vi "Read Tag Data.vi"(8 "error in (no error)":errorcluster, 11 "Task D-O Channels":string[][](array[string])) -> (0 "error out":errorcluster, 3 "Array":bool[][](array[boolean]))   [LabVIEW 2018, in "DAQ.lvlib"]
uses:
  DAQ.lvlib
  Tag VIs/Tag FGV Operation Enum.ctl
  Shared Variables/Dynamic Shared Variables.lvlib
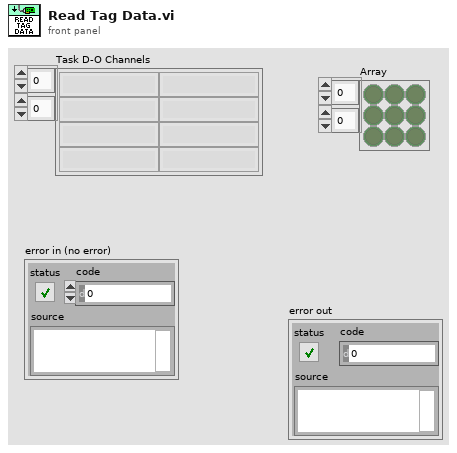
[diagram p1: front panel]
types:
  T1 = typedef "Tag FGV Operation Enum.ctl" = enum16{"Init", "Set Notification Queue", "Create Tag", "Commit", "Write Tag (Numeric)", "Write Tag (Boolean)", "Read All Tags", "Read One Tag", "Delete Tag Category", "Set Alarm Parameters (Numeric)", "Set Alarm Parameters (Boolean)", "Enable All Alarms", "Disable All Alarms", "Delete All Tags", "Read Alarms", "Ack Alarm"}
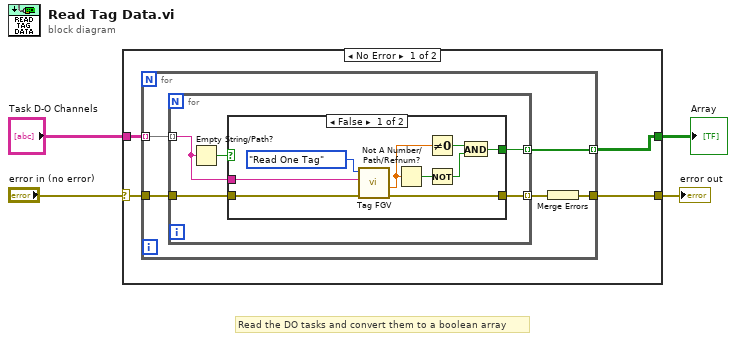
[diagram p0: block diagram]
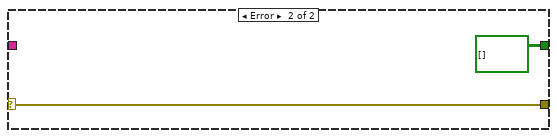
[diagram p3: hidden frame]
diagram:
  # "Read the DO tasks and convert them to a boolean array"
  n1 = case shown="No Error" "error in (no error)" {
    selector: "error in (no error)" -> [w6 w30]
    tunnel: [w8 w30] -> w4
    tunnel: "Task D-O Channels" -> [w7 _]
    tunnel: [w5 bool[][] []] -> w2
    frame No Error {
      n2 = for {
        tunnel: [w13] -> w8
        tunnel: w7 -> [w9] mode=indexing
        tunnel: w6 -> [w11]
        tunnel: [w10] -> w5 mode=indexing
        n3 = for {
          tunnel: [w16] -> w10 mode=indexing
          tunnel: w9 -> [w14] mode=indexing
          tunnel: w11 -> [w18]
          tunnel: [w17] -> w12 mode=indexing
          n4 = Empty String/Path?(string/path=w14) -> (empty?=w15:bool)
          n5 = case shown="False" w15 {
            tunnel: w14 -> [w26 _]
            tunnel: w18 -> [w25 w28]
            tunnel: [w24 w28] -> w17
            tunnel: [w22 _] -> w16
            frame False {
              n6 = call "Tag FGV.vi"("error in (no error)"=w25, "Tag Name"=w26, "Operation"=Tag_FGV_Operation_Enum."Read One Tag") -> ("error out"=w24:errorcluster, "Tag Value"=w21:dbl)  [unwired: 3 in, 4 out]
              n7 = Not A Number/Path/Refnum?(number/path/refnum=w21) -> (NaN/Path/Refnum?=w20:bool)
              n8 = Not Equal To 0?(x=w21) -> (x != 0?=w23:bool)
              n9 = Not(x=w20) -> (.not. x?=w19:bool)
              n10 = And(x=w23, y=w19) -> (x .and. y?=w22:bool)
            }
            frame True {
            }
          }
        }
        n11 = Merge Errors(w12) -> (w13:errorcluster)
      }
    }
    frame Error {
    }
  }
  "error out" <- w4
  "Array" <- w2
